vi "Get SLSC Switch Info.vi"(8 "error in (no error)":errorcluster, 10 "relay string":string, 11 "SLSC Switch in":refnum<class "SLSC Switch.lvclass">) -> (0 "error out":errorcluster, 2 "SLSC Switch Info":T1, 3 "SLSC Switch out":refnum<class "SLSC Switch.lvclass">)   [LabVIEW 2015, in "SLSC Switch.lvclass"]
uses:
  SLSC Switch.lvclass
  Controls/SLSC Relay Info.ctl
  SLSC Switch.lvclass/SLSC Switch.ctl
  Route Manager/Route Manager.lvclass
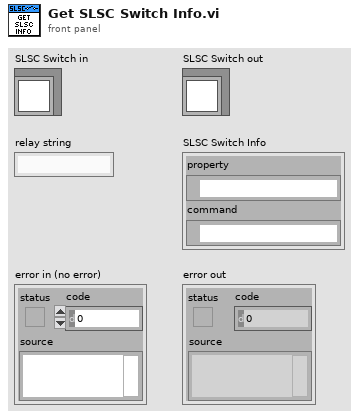
[diagram p1: front panel]
types:
  T1 = typedef "SLSC Switch.lvclass/SLSC Relay Info.ctl" = cluster{"property":refnum<k21>, "command":refnum<k21>}
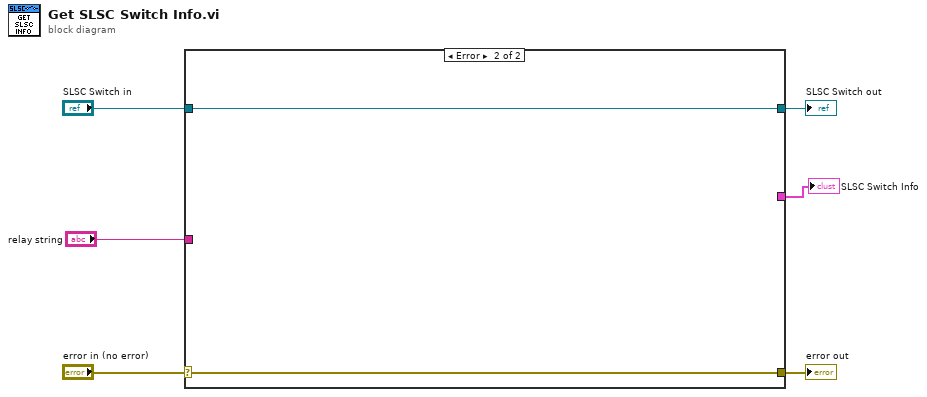
[diagram p0: block diagram]
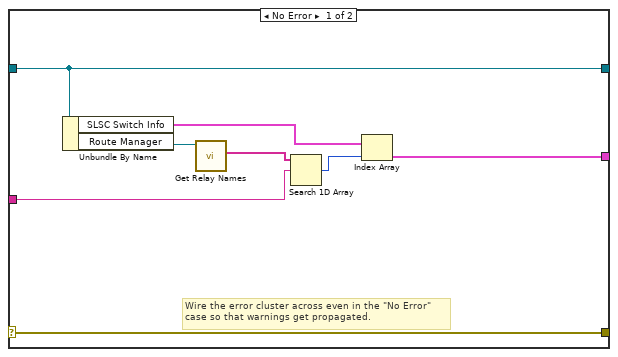
[diagram p2: hidden frame]
diagram:
  n1 = case shown="Error" "error in (no error)" {
    selector: "error in (no error)" -> [w14 w16]
    tunnel: [w14 w16] -> w5
    tunnel: [w13 w15] -> w3
    tunnel: "SLSC Switch in" -> [w13 w15]
    tunnel: "relay string" -> [w10 _]
    tunnel: [w7 _] -> w1
    frame No Error {
      # "Wire the error cluster across even in the \"No Error\"\ncase so that warnings get propagated."
      n2 = Unbundle By Name(w13) -> ("SLSC Switch Info"=w9:T1[], "Route Manager"=w12:refnum<class "Route Manager.lvclass">)
      n3 = call "Get Relay Names.vi"("Route Manager in"=w12) -> ("relay strings"=w11:string[])  [unwired: 8 in, 2 out]
      n4 = Search 1D Array(1D array=w11, element=w10) -> (index of element=w8:i32)  [unwired: 1 in]
      n5 = Index Array(array=w9, index=w8) -> (element=w7:T1)
    }
    frame Error {
    }
  }
  "error out" <- w5
  "SLSC Switch out" <- w3
  "SLSC Switch Info" <- w1
